vi "RT Errors.To String.Integer.Decimal.U8.vi"(1 "value":u8) -> (0 "value as string":string)   [LabVIEW 2016, in "RT Error Handling.lvlib"]
doc: "Converts the provided <B>value</B> into a decimal-formatted string."
uses:
  RT Error Handling.lvlib
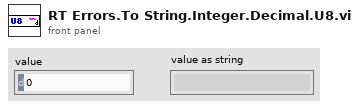
[diagram p1: front panel]
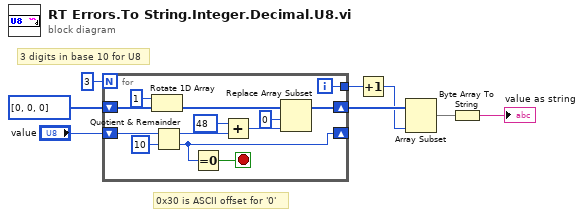
[diagram p0: block diagram]
diagram:
  # "0x30 is ASCII offset for '0'"
  # "3 digits in base 10 for U8"
  n1 = for {
    N: 3 -> [_]
    shift-right: [w20] -> w4
    shift-left: u8[] [0, 0, 0] -> [w12]
    shift-right: [w15] -> _
    shift-left: "value" -> [w17]
    tunnel: [w9] -> w2
    i -> [w9]
    stop <- w14 stop-if-true
    n2 = Rotate 1D Array(1:w12, 2:1 ("n")) -> (0:w11:u8[])
    n3 = Quotient & Remainder(x=w17, y=u8 10) -> (x-y*floor(x/y)=w16:u8, floor(x/y)=w15:u8)
    n4 = Equal To 0?(x=w15) -> (x = 0?=w14:bool)
    n5 = Add(x=u8 48 ("y"), y=w16) -> (x+y=w21:u8)
    n6 = Replace Array Subset(array=w11, new element=w21, index=0) -> (w20:u8[])
  }
  n7 = Increment(x=w2) -> (x+1=w1:i32)
  n8 = Array Subset(array=w4, length=w1) -> (w3:u8[])  [unwired: 1 in]
  n9 = Byte Array To String(unsigned byte array=w3) -> (string=→"value as string":string)
